vi "ReadBatteryCurve.vi"() -> (2 "subarray 2":dbl[](array[numeric]))   [LabVIEW 2021]
uses:
  <vilib>/Utility/file.llb/Read Delimited Spreadsheet (DBL).vi
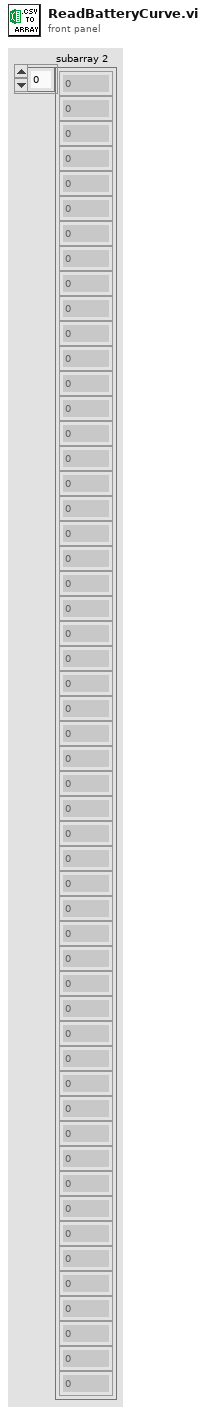
[diagram p1: front panel]
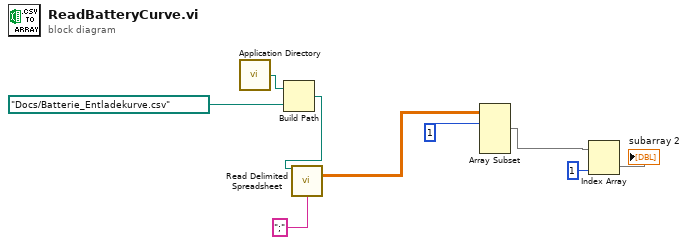
[diagram p0: block diagram]
diagram:
  n1 = call <vilib>:"Application Directory.vi"() -> ("Application Directory"=w5:path)
  n2 = Build Path(base path=w5, name or relative path=path "Docs/Batterie_Entladekurve.csv") -> (appended path=w6:path)
  n3 = call-poly <vilib>:"Read Delimited Spreadsheet.vi"("file path (dialog if empty)"=w6, "delimiter (\\t)"=";" ("delimiter (\\t)")) -> ("all rows"=w8:dbl[][])  [unwired: 8 in, 5 out]
  n4 = Array Subset(array=w8, index (row)=1 ("index")) -> (w3:dbl[][])  [unwired: 3 in]
  n5 = Index Array(array=w3, index (col)=1 ("disabled index (col)")) -> (element=→"subarray 2":dbl[])  [unwired: 1 in]
